vi "CreateHTML.vi"(0 "WebFrontPanel":refnum<class "WebFrontPanel.lvclass">, 1 "Refresh rate (250ms)":i32=250, 5 "error in (no error)":errorcluster) -> (19 "error out":errorcluster)   [LabVIEW 2014, in "FrontPanelPublisher.lvlib" / "FrontPanelManager.lvclass"]
uses:
  FrontPanelManager.lvclass
  WebFrontPanel_class/WebFrontPanel.lvclass
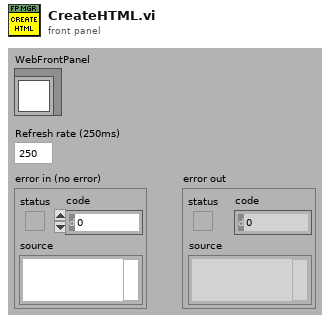
[diagram p1: front panel]
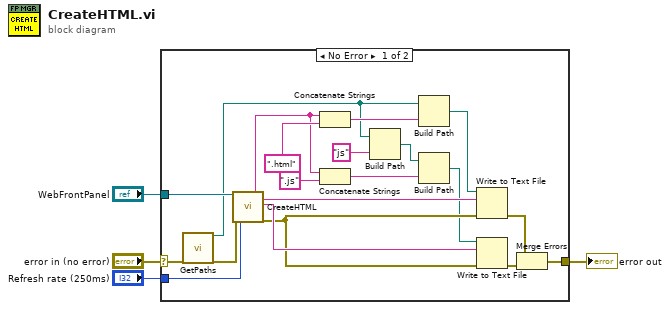
[diagram p0: block diagram]
diagram:
  n1 = case shown="No Error" "error in (no error)" {
    selector: "error in (no error)" -> [w6 w25]
    tunnel: [w12 w25] -> w3
    tunnel: "WebFrontPanel" -> [w24 _]
    tunnel: "Refresh rate (250ms)" -> [w8 _]
    frame No Error {
      n2 = call "GetPaths.vi"("error in (no error)"=w6) -> ("Root folder"=w7:path, "error out"=w5:errorcluster)  [unwired: 15 in, 2 out]
      n3 = call-dynamic "CreateHTML.vi"("reference in"=w24, "error in (no error)"=w5, "Refresh rate (250ms)"=w8) -> ("Name"=w22:string, "HTML"=w18:string, "js"=w16:string, "error out"=w15:errorcluster)  [unwired: 12 in, 1 out]
      n4 = Concatenate Strings(w22, ".html") -> (w19:string)
      n5 = Concatenate Strings(w22, ".js") -> (w20:string)
      n6 = Build Path(base path=w7, name or relative path="js") -> (appended path=w10:path)
      n7 = Build Path(base path=w7, name or relative path=w19) -> (appended path=w17:path)
      n8 = Build Path(base path=w10, name or relative path=w20) -> (appended path=w9:path)
      n9 = Write to Text File(file (use dialog)=w17, text=w18, error in=w15) -> (error out=w13:errorcluster)  [unwired: 1 in, 2 out]
      n10 = Write to Text File(file (use dialog)=w9, text=w16, error in=w15) -> (error out=w14:errorcluster)  [unwired: 1 in, 2 out]
      n11 = Merge Errors(w13, w14) -> (w12:errorcluster)
    }
    frame Error {
    }
  }
  "error out" <- w3
